vi "Convert U64 Data to Image.vi"(7 "Image Data":u64[](array[numeric]), 8 "error in":errorcluster, 9 "Image Width":u32, 10 "Image Height":u32, 11 "Image Destination In":T1) -> (0 "error out":errorcluster, 3 "Image Destination Out":T1)   [LabVIEW 2013]
uses:
  <vilib>/vision/Image Controls.llb/IMAQ Image.ctl
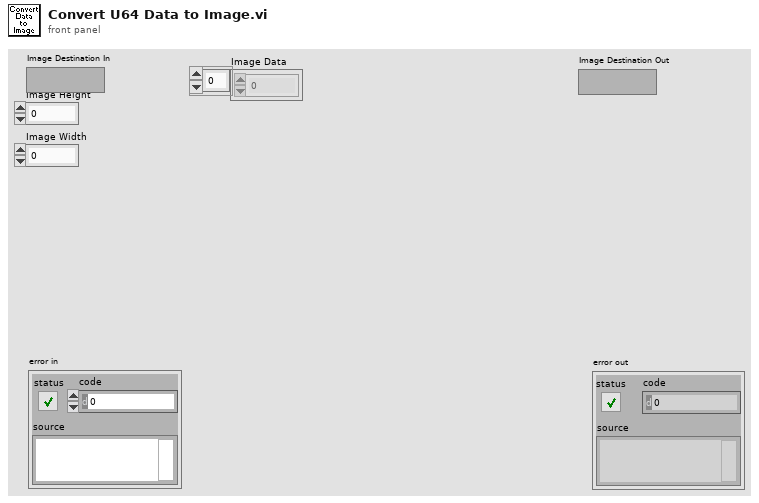
[diagram p1: front panel]
types:
  T1 = typedef "IMAQ Image.ctl" = refnum<image>
  T2 = enum16{"big-endian, network order", "native, host order", "little-endian"}
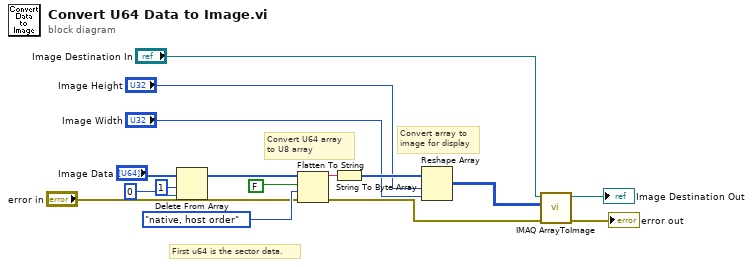
[diagram p0: block diagram]
diagram:
  # "First u64 is the sector data."
  # "Convert U64 array\nto U8 array"
  # "Convert array to\nimage for display"
  n1 = Delete From Array(array="Image Data", length=1, index=0) -> (array with subset deleted=w3:u64[])  [unwired: 1 out]
  n2 = Flatten To String(anything=w3, prepend array or string size? (T)=FALSE, byte order (0:big-endian, network order)=T2."native, host order", error in (no error)="error in") -> (data string=w13:string, error out=w6:errorcluster)  [unwired: 1 out]
  n3 = String To Byte Array(string=w13) -> (unsigned byte array=w12:u8[])
  n4 = Reshape Array(w12, "Image Height", "Image Width") -> (w16:u8[][])
  n5 = call "IMAQ ArrayToImage"("error in (no error)"=w6, "Image Pixels (U8)"=w16, "Image"="Image Destination In") -> ("error out"=→"error out":errorcluster, "Image Out"=→"Image Destination Out":T1)  [unwired: 7 in]
